vi "test New And Old Values Match.vi"(8 "error in (no error)":errorcluster, 11 "TestCase in":refnum<class "Routing and Faulting Aliases Unit Tests.lvclass">) -> (0 "error out":errorcluster, 3 "TestCase out":refnum<class "Routing and Faulting Aliases Unit Tests.lvclass">)   [LabVIEW 2020, in "Routing and Faulting Aliases Unit Tests.lvclass"]
uses:
  Routing and Faulting Aliases Unit Tests.lvclass
  Shared/Alias Mapping.ctl
  Shared/Alias Endpoint.ctl
  System Explorer/Alias.ctl
  System Explorer/Endpoint.ctl
  Routing and Faulting Aliases Unit Tests.lvclass/Routing and Faulting Aliases Unit Tests.ctl
  <vilib>/addons/_JKI Toolkits/VI Tester/TestCase.llb/TestCase.lvclass
  System Explorer/Routing and Faulting System Explorer.lvlib
  Scripting/Routing and Faulting Scripting.lvlib
  Shared/Routing and Faulting Shared.lvlib
  C:/Program Files (x86)/National Instruments/LabVIEW 2020/vi.lib/addons/_JKI Toolkits/VI Tester/TestCase.llb/TestCase.lvclass
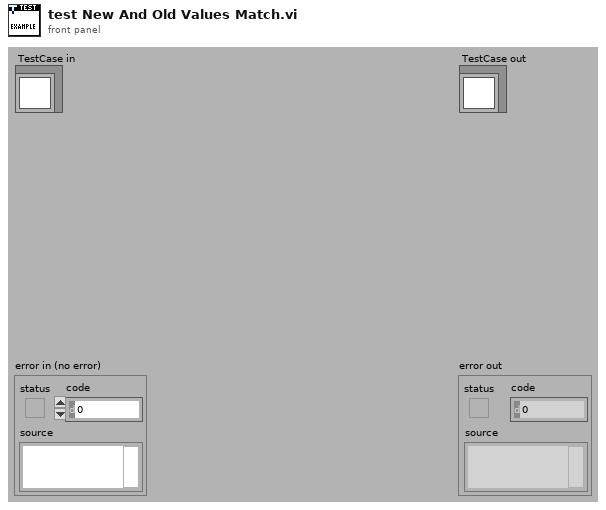
[diagram p1: front panel]
types:
  T1 = typedef "Routing and Faulting System Explorer.lvlib/Endpoint.ctl" = string
  T2 = typedef "Routing and Faulting System Explorer.lvlib/Alias.ctl" = cluster{"Endpoint":T1, "Alias":string, "Remove":bool}
  T3 = typedef "Routing and Faulting Shared.lvlib/Alias Mapping.ctl" = cluster{"Alias":string, "Endpoint":T4}
  T4 = typedef "Routing and Faulting Shared.lvlib/Alias Endpoint.ctl" = cluster{"Module Path":string, "Endpoint":string}
  T5 = typedef "Custom Device API.lvlib/Custom Device Item Ref.ctl" = u64
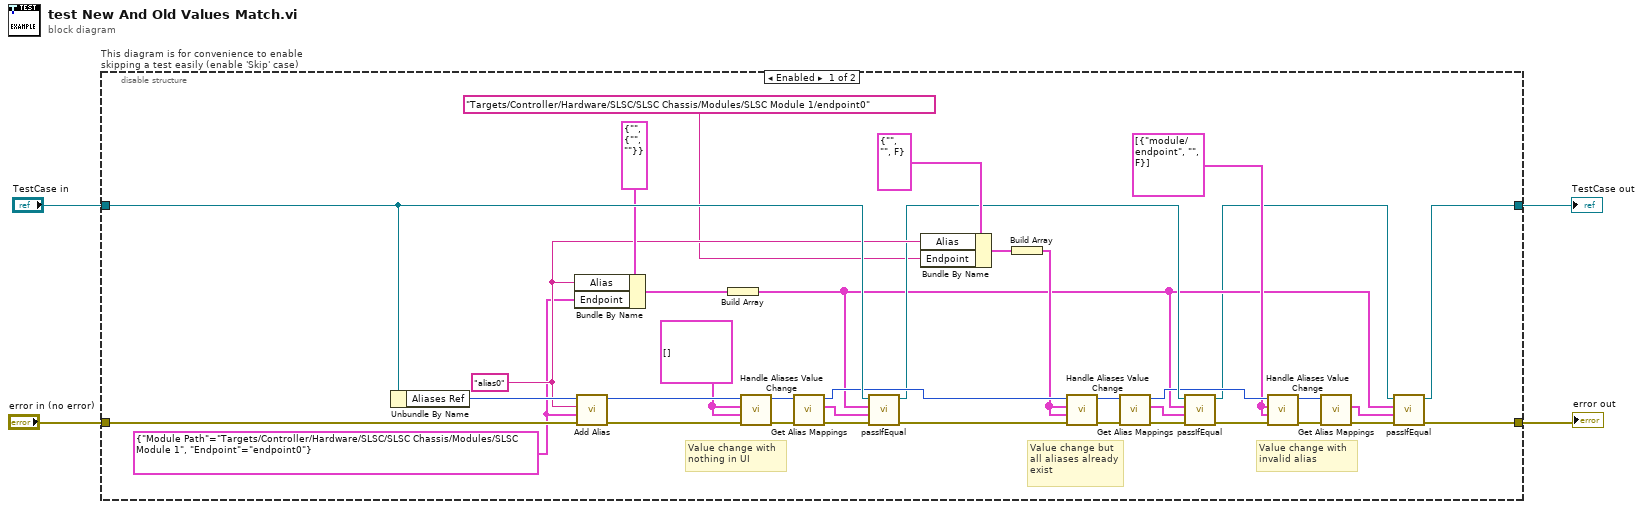
[diagram p0: block diagram]
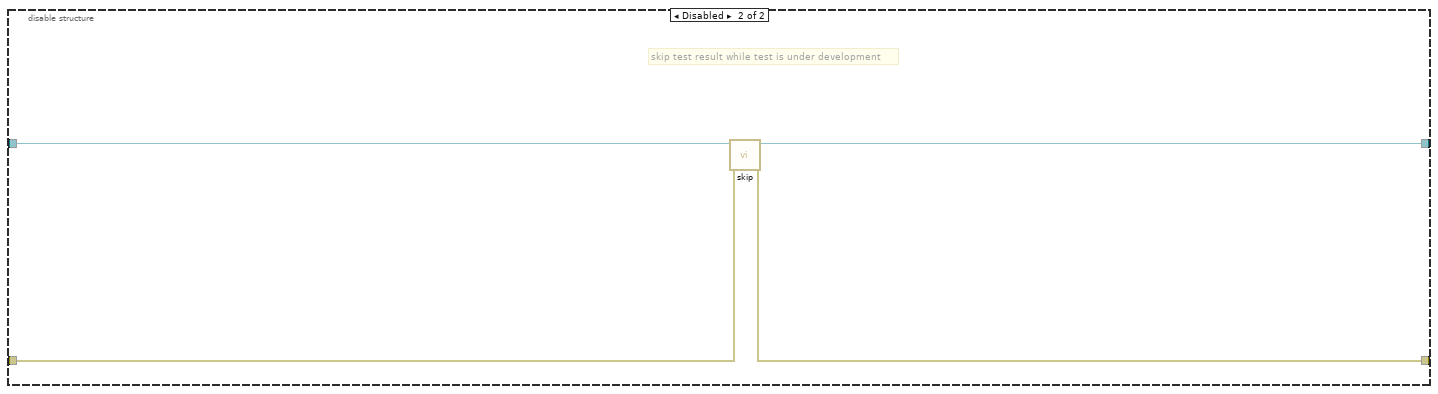
[diagram p2: hidden frame]
diagram:
  n1 = disable-structure "This diagram is for convenience to enable skipping a test easily (enable 'Skip' case)" shown="Enabled" {
    disable-tunnel: "TestCase in" -> [w37 w44]
    disable-tunnel: [w8 w42] -> w1
    disable-tunnel: [w7 w43] -> w3
    disable-tunnel: "error in (no error)" -> [w36 w41]
    frame Enabled {
      w6 = T4 {"Module Path"="Targets/Controller/Hardware/SLSC/SLSC Chassis/Modules/SLSC Module 1", "Endpoint"="endpoint0"} ("Endpoint")
      w14 = T2[] [{"Endpoint"="module/endpoint", "Alias"="", "Remove"=FALSE}] ("appended array")
      w31 = T2[] [] ("NewVal")
      w26 = "alias0" ("Alias")
      # "Value change with\ninvalid alias"
      # "Value change but\nall aliases already\nexist"
      # "Value change with\nnothing in UI"
      n2 = Unbundle By Name(w37) -> ("Aliases Ref"=w35:T5)
      n3 = Bundle By Name(cluster=T3 {"Alias"="", "Endpoint"={"Module Path"="", "Endpoint"=""}} ("Alias Mapping"), "Alias"=w26, "Endpoint"=w6) -> (w18:T3)
      n4 = call "Add Alias.vi"("error in"=w36, "endpoint"=w6, "alias"=w26, "endpoint aliases in"=w35) -> ("error out"=w34:errorcluster, "endpoint aliases out"=w33:T5)  [unwired: 6 in]
      n5 = Build Array(w18) -> (w11:T3[])
      n6 = call "Handle Aliases Value Change.vi"("error in (no error)"=w34, "OldVal"=w31, "NewVal"=w31, "Aliases Ref in"=w33) -> ("error out"=w40:errorcluster, "Aliases Ref out"=w39:T5)  [unwired: 4 in, 2 out]
      n7 = call "Get Alias Mappings.vi"("error in"=w40, "endpoint aliases in"=w39) -> ("error out"=w38:errorcluster, "alias mappings"=w30:T3[], "endpoint aliases out"=w28:T5)  [unwired: 7 in]
      n8 = call-dynamic "passIfEqual.vi"("error in (no error)"=w38, "y"=w30, "x"=w11, "TestCase in"=w37) -> ("error out"=w29:errorcluster, "TestCase out"=w23:refnum<class "Routing and Faulting Aliases Unit Tests.lvclass">)  [unwired: 6 in]
      n9 = Bundle By Name(cluster=T2 {"Endpoint"="", "Alias"="", "Remove"=FALSE} ("Alias"), "Alias"=w26, "Endpoint"=T1 "Targets/Controller/Hardware/SLSC/SLSC Chassis/Modules/SLSC Module 1/endpoint0") -> (w25:T2)
      n10 = Build Array(w25) -> (w24:T2[])
      n11 = call "Handle Aliases Value Change.vi"("error in (no error)"=w29, "OldVal"=w24, "NewVal"=w24, "Aliases Ref in"=w28) -> ("error out"=w22:errorcluster, "Aliases Ref out"=w21:T5)  [unwired: 4 in, 2 out]
      n12 = call "Get Alias Mappings.vi"("error in"=w22, "endpoint aliases in"=w21) -> ("error out"=w20:errorcluster, "alias mappings"=w19:T3[], "endpoint aliases out"=w15:T5)  [unwired: 7 in]
      n13 = call-dynamic "passIfEqual.vi"("error in (no error)"=w20, "y"=w19, "x"=w11, "TestCase in"=w23) -> ("error out"=w16:errorcluster, "TestCase out"=w9:refnum<class "Routing and Faulting Aliases Unit Tests.lvclass">)  [unwired: 6 in]
      n14 = call "Handle Aliases Value Change.vi"("error in (no error)"=w16, "OldVal"=w14, "NewVal"=w14, "Aliases Ref in"=w15) -> ("error out"=w17:errorcluster, "Aliases Ref out"=w13:T5)  [unwired: 4 in, 2 out]
      n15 = call "Get Alias Mappings.vi"("error in"=w17, "endpoint aliases in"=w13) -> ("error out"=w12:errorcluster, "alias mappings"=w10:T3[])  [unwired: 7 in, 1 out]
      n16 = call-dynamic "passIfEqual.vi"("error in (no error)"=w12, "y"=w10, "x"=w11, "TestCase in"=w9) -> ("error out"=w7:errorcluster, "TestCase out"=w8:refnum<class "Routing and Faulting Aliases Unit Tests.lvclass">)  [unwired: 6 in]
    }
    frame Disabled {
      # "skip test result while test is under development"
      n17 = call <vilib>:"skip.vi"("error in (no error)"=w41, "TestCase in"=w44) -> ("error out"=w43:errorcluster, "TestCase out"=w42:refnum<class "Routing and Faulting Aliases Unit Tests.lvclass">)  [unwired: 8 in]
    }
  }
  "error out" <- w3
  "TestCase out" <- w1
